vi "H5close.vi"(3 "dtype_id":i32, 9 "error in (no error)":errorcluster) -> (0 "status":i32, 6 "error out":errorcluster)   [LabVIEW 2009]
uses:
  hdf5dll.dll
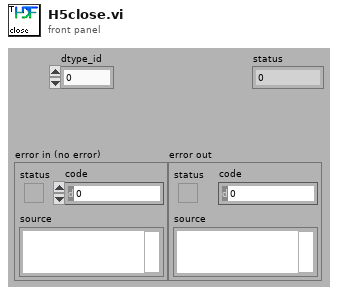
[diagram p1: front panel]
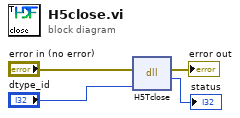
[diagram p0: block diagram]
diagram:
  n1 = dll-call lib="hdf5dll.dll" fn="H5Tclose"(error in="error in (no error)", "dtype_id"="dtype_id") -> (error out=→"error out":errorcluster, "return type"=→"status":i32)  [unwired: 3 in, 1 out]
